vi "robotic arm main.vi"() -> ()   [LabVIEW 2019]
uses:
  <vilib>/myRIO/Instrument Drivers/Onboard IO/DIO/typedefs/DIO Reference.ctl
  <vilib>/myRIO/Common/Instrument Driver Framework/Utilities/typedefs/myRIO Generic Hardware Reference.ctl
  <vilib>/myRIO/Common/Instrument Driver Framework/Utilities/typedefs/Hardware Version Enum.ctl
  <vilib>/myRIO/Common/Instrument Driver Framework/Utilities/typedefs/myRIO v1.0 Reference.ctl
  <vilib>/myRIO/Common/Instrument Driver Framework/Utilities/typedefs/Generic FPGA Reference.ctl
  <vilib>/myRIO/Common/Instrument Driver Framework/myRIO v1.0/DIO/typedefs/DIO Channels List.ctl
  <vilib>/myRIO/Common/Instrument Driver Framework/myRIO v1.0/DIO/typedefs/DIO Channels Enum.ctl
  <vilib>/userdefined/High Color/nirio_resource_hc.ctl
  <vilib>/myRIO/Instrument Drivers/Onboard IO/PWM/typedefs/PWM Reference.ctl
  <vilib>/myRIO/Common/Instrument Driver Framework/myRIO v1.0/PWM/typedefs/PWM Channels Enum.ctl
  <vilib>/myRIO/Instrument Drivers/Onboard IO/PWM/typedefs/PWM Configuration.ctl
  <vilib>/myRIO/Common/Instrument Driver Framework/Utilities/vis/Is FPGA Ref Available.vi
  <vilib>/myRIO/Common/Instrument Driver Framework/myRIO v1.0/DIO/vis/myRIO v1.1 Open DIO.vi
  <vilib>/myRIO/Instrument Drivers/Onboard IO/DIO/vis/Read.vi
  <vilib>/myRIO/Common/Instrument Driver Framework/myRIO v1.0/PWM/vis/myRIO v1.1 Open PWM.vi
  <vilib>/myRIO/Instrument Drivers/Onboard IO/PWM/vis/Set Duty Cycle and Frequency.vi
  <vilib>/myRIO/Common/Instrument Driver Framework/Utilities/vis/Validate Channels.vi
  <vilib>/myRIO/Common/Instrument Driver Framework/myRIO v1.0/DIO/vis/myRIO v1.0 Reserve DIO.vi
  <vilib>/myRIO/Common/Instrument Driver Framework/myRIO v1.0/PWM/vis/myRIO v1.0 Reserve PWM.vi
  <vilib>/myRIO/Common/Instrument Driver Framework/myRIO v1.0/Resource Manager/vis/myRIO v1.0 Reserve Channel List.vi
  <vilib>/myRIO/Common/Instrument Driver Framework/myRIO v1.0/DIO/vis/myRIO v1.0 Build MUX Configuration DIO.vi
  <vilib>/myRIO/Common/Instrument Driver Framework/myRIO v1.0/PWM/vis/myRIO v1.0 Build MUX Configuration PWM.vi
  <vilib>/myRIO/Common/Instrument Driver Framework/myRIO v1.0/Resource Manager/vis/myRIO v1.0 Reserve Channel.vi
  <vilib>/myRIO/Common/Instrument Driver Framework/myRIO v1.0/Resource Manager/vis/myRIO v1.0 Unreserve Channel.vi
  <vilib>/myRIO/Common/Instrument Driver Framework/myRIO v1.0/Resource Manager/vis/myRIO v1.0 Create Configuration List.vi
  <vilib>/myRIO/Common/Instrument Driver Framework/myRIO v1.0/Resource Manager/vis/myRIO v1.0 Build Mutex Name.vi
  <vilib>/Utility/VariantDataType/GetNumericInfo.vi
  <vilib>/Utility/error.llb/Error Cluster From Error Code.vi
  <vilib>/myRIO/Common/Instrument Driver Framework/myRIO v1.0/myRIO v1.1 Open.vi
  <vilib>/myRIO/Common/Instrument Driver Framework/Utilities/vis/IO Manager.vi
  <vilib>/myRIO/Common/Instrument Driver Framework/Utilities/vis/Configuration Manager.vi
  <vilib>/myRIO/Common/Instrument Driver Framework/myRIO v1.0/Resource Manager/vis/myRIO v1.0 Configure IO.vi
  <vilib>/myRIO/Common/Instrument Driver Framework/myRIO v1.0/myRIO v1.0 Close.vi
  <vilib>/myRIO/Common/Instrument Driver Framework/myRIO v1.0/DIO/vis/myRIO v1.0 Read DIO.vi
  <vilib>/myRIO/Common/Instrument Driver Framework/myRIO v1.0/PWM/vis/myRIO v1.0 Write PWM.vi
  <vilib>/robotics/Kinematics/Generate Joint Trajectory (Int).vi
  <vilib>/myRIO/Express VI/Onboard IO/DI/DI Express VI.xnode
  <vilib>/myRIO/Instrument Drivers/Onboard IO/DIO/vis/myRIO DIO Open.xnode
  <vilib>/myRIO/Express VI/Onboard IO/PWM/PWM Express VI.xnode
  <vilib>/myRIO/Instrument Drivers/Onboard IO/PWM/vis/myRIO PWM Open.xnode
  <vilib>/robotics/Kinematics/NI_Kinematics.lvlib
  <vilib>/myRIO/Instrument Drivers/Onboard IO/PWM/PWM.lvlib
  <vilib>/myRIO/Instrument Drivers/Onboard IO/DIO/DIO.lvlib
panel:
  out "Position Sensor 2 (Pin 13)":bool
  out "Position Sensor 1 (Pin 11)":bool
  in  "Motion sequence or predefined?":bool
  out "State Number":i32
  in  "Motion sequence":T1
  in  "Control 6":dbl
  in  "Control 5":dbl
  in  "Control 4":dbl
  in  "Control 3":dbl
  in  "Control 2":dbl
  in  "Control 1":dbl
  out "1":dbl
  out "2":dbl
  out "3":dbl
  out "4":dbl
  out "5":dbl
  out "6":dbl
  in  "Start (Press time to start the action)":bool
  out "transposed array":dbl[][](array[numeric])
  out "start position":i32[](array[numeric])
  out "end position":i32[](array[numeric])
  out "joint position trajectory":dbl[][](array[numeric])
  out "Servo 1":dbl[](graph)
  out "Angle 1":dbl
  out "Angle 2":dbl
  out "Angle 3":dbl
  out "Angle 4":dbl
  out "Angle 5":dbl
  out "Angle 6":dbl
  out "Servo 2":dbl[](graph)
  out "Servo 3":dbl[](graph)
  out "Servo 4":dbl[](graph)
  out "Servo 5":dbl[](graph)
  out "Servo 6":dbl[](graph)
  in  "Switch mode":bool
  # "Agriculture Phenotyping Automation"
  # "EEM323 Robotics 2023\nMini Project Group 4\nLai Hong You, Justin Chia Vern Shuen, Thow Zhi An, Tiong Ji Kai"
  # "Control"
  # "Trajectory and Servos Status"
  # "State machine status"
  # "Motion \nSequence"
  # "Predefined"
  # "Sensor"
  # "Manual"
  # "Input"
  # "Output"
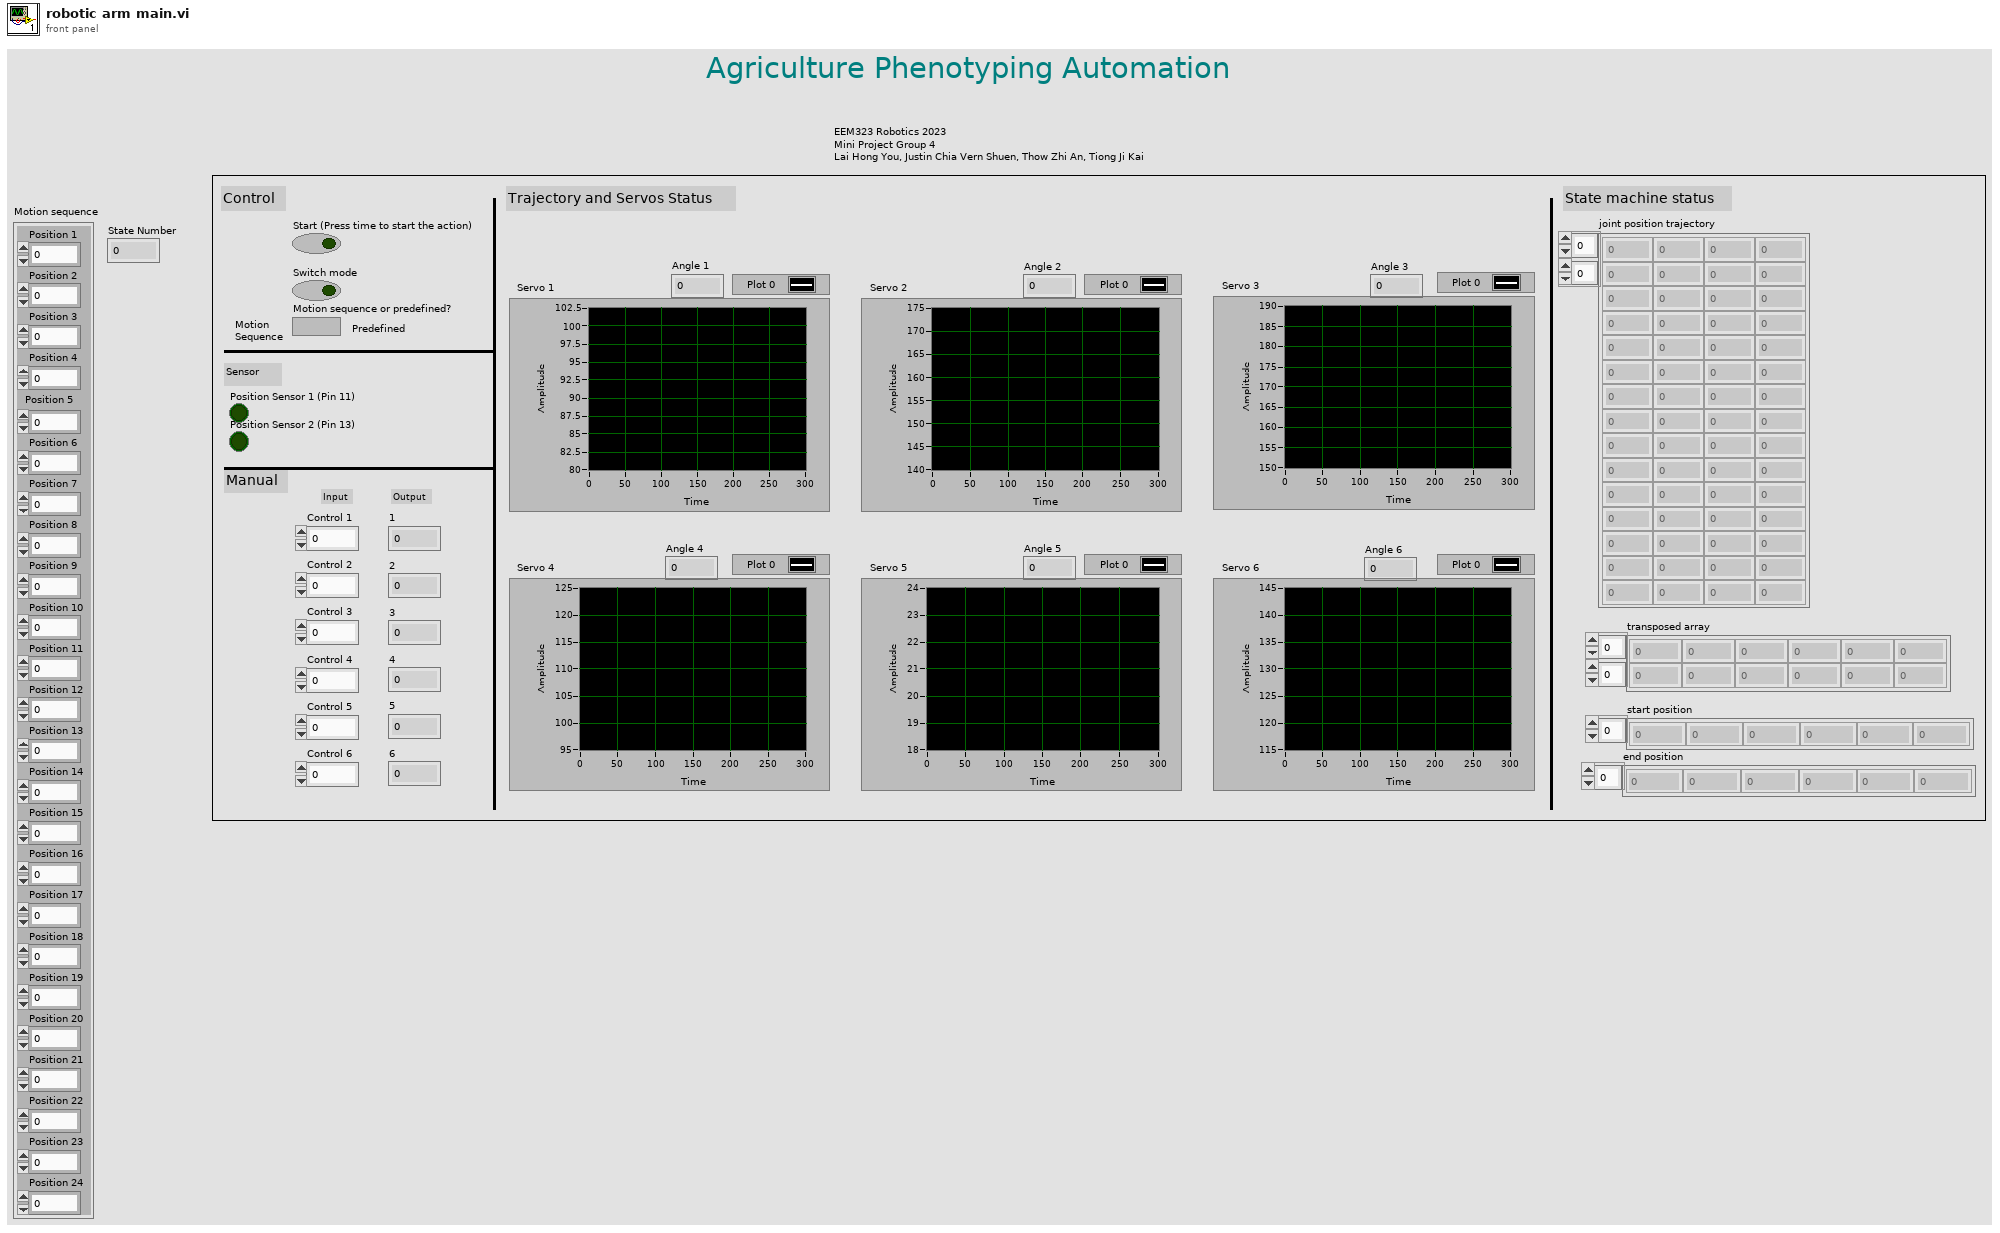
[diagram p1: front panel]
types:
  T1 = cluster{"Position 1":dbl, "Position 2":dbl, "Position 3":dbl, "Position 4":dbl, "Position 5":dbl, "Position 6":dbl, "Position 7":dbl, "Position 8":dbl, "Position 9":dbl, "Position 10":dbl, "Position 11":dbl, "Position 12":dbl, "Position 13":dbl, "Position 14":dbl, "Position 15":dbl, "Position 16":dbl, "Position 17":dbl, "Position 18":dbl, "Position 19":dbl, "Position 20":dbl, "Position 21":dbl, "Position 22":dbl, "Position 23":dbl, "Position 24":dbl}
  T2 = typedef "PWM.lvlib/PWM Reference.ctl" = cluster{"myRIO Reference":T3, "PWM Channels Enum":T7, "PWM Configuration":T8}
  T3 = typedef "myRIO Generic Hardware Reference.ctl" = cluster{"myRIO Model":T4, "myRIO Hardware Reference":T5}
  T4 = typedef "Hardware Version Enum.ctl" = enum16{"Unknown", "myRIO-1900", "myRIO-1950", "roboRIO", "NI ELVIS RIO CM", "ELVIS III"}
  T5 = typedef "myRIO v1.0 Reference.ctl" = cluster{"Generic FPGA Reference":T6, "Allow multiple opens":bool}
  T6 = typedef "Generic FPGA Reference.ctl" = refnum<k20>
  T7 = typedef "PWM Channels Enum.ctl" = enum16{"Not Connected", "C/PWM0", "C/PWM1", "A/PWM0", "A/PWM1", "A/PWM2", "A/PWM3", "A/PWM4", "A/PWM5", "A/PWM6", "A/PWM7", "A/PWM8", "A/PWM9", "A/PWM10", "A/PWM11", "A/PWM12", "A/PWM13", "A/PWM14", "A/PWM15", "A/PWM16", "A/PWM17", "A/PWM18", "A/PWM19", "B/PWM0", "B/PWM1", "B/PWM2", "B/PWM3", "B/PWM4", "B/PWM5", "B/PWM6", "B/PWM7", "B/PWM8", "B/PWM9", "B/PWM10", "B/PWM11", "B/PWM12", "B/PWM13", "B/PWM14", "B/PWM15", "B/PWM16", "B/PWM17", "B/PWM18", "B/PWM19", "PWM/PWM0", "PWM/PWM1", "PWM/PWM2", "PWM/PWM3", "PWM/PWM4", "PWM/PWM5", "PWM/PWM6", "PWM/PWM7", "PWM/PWM8", "PWM/PWM9"}
  T8 = typedef "PWM.lvlib/PWM Configuration.ctl" = cluster{"Frequency":dbl, "Duty Cycle":dbl}
  T9 = typedef "nirio_resource_hc.ctl" = tag
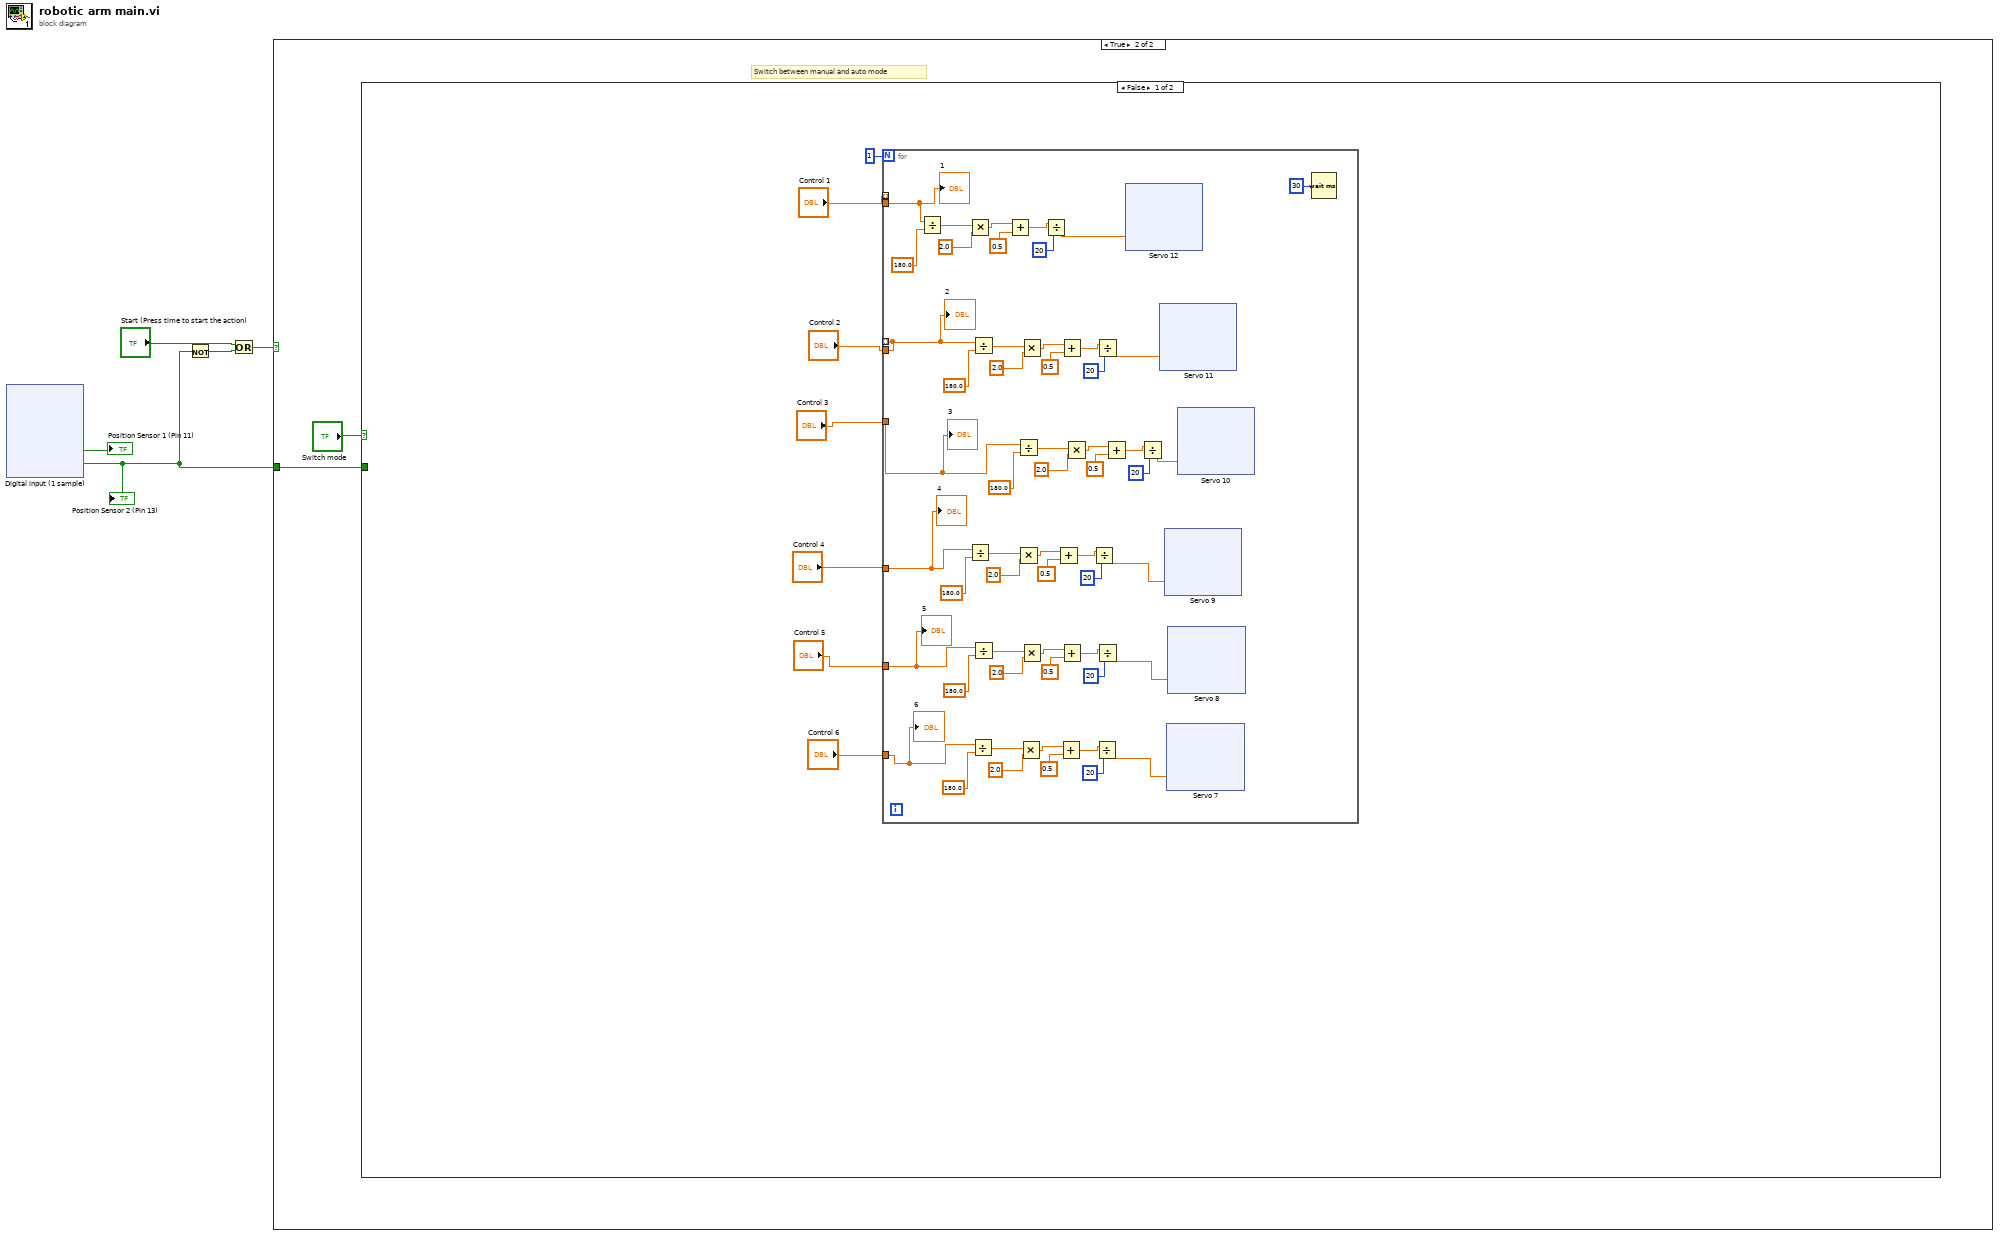
[diagram p0: block diagram]
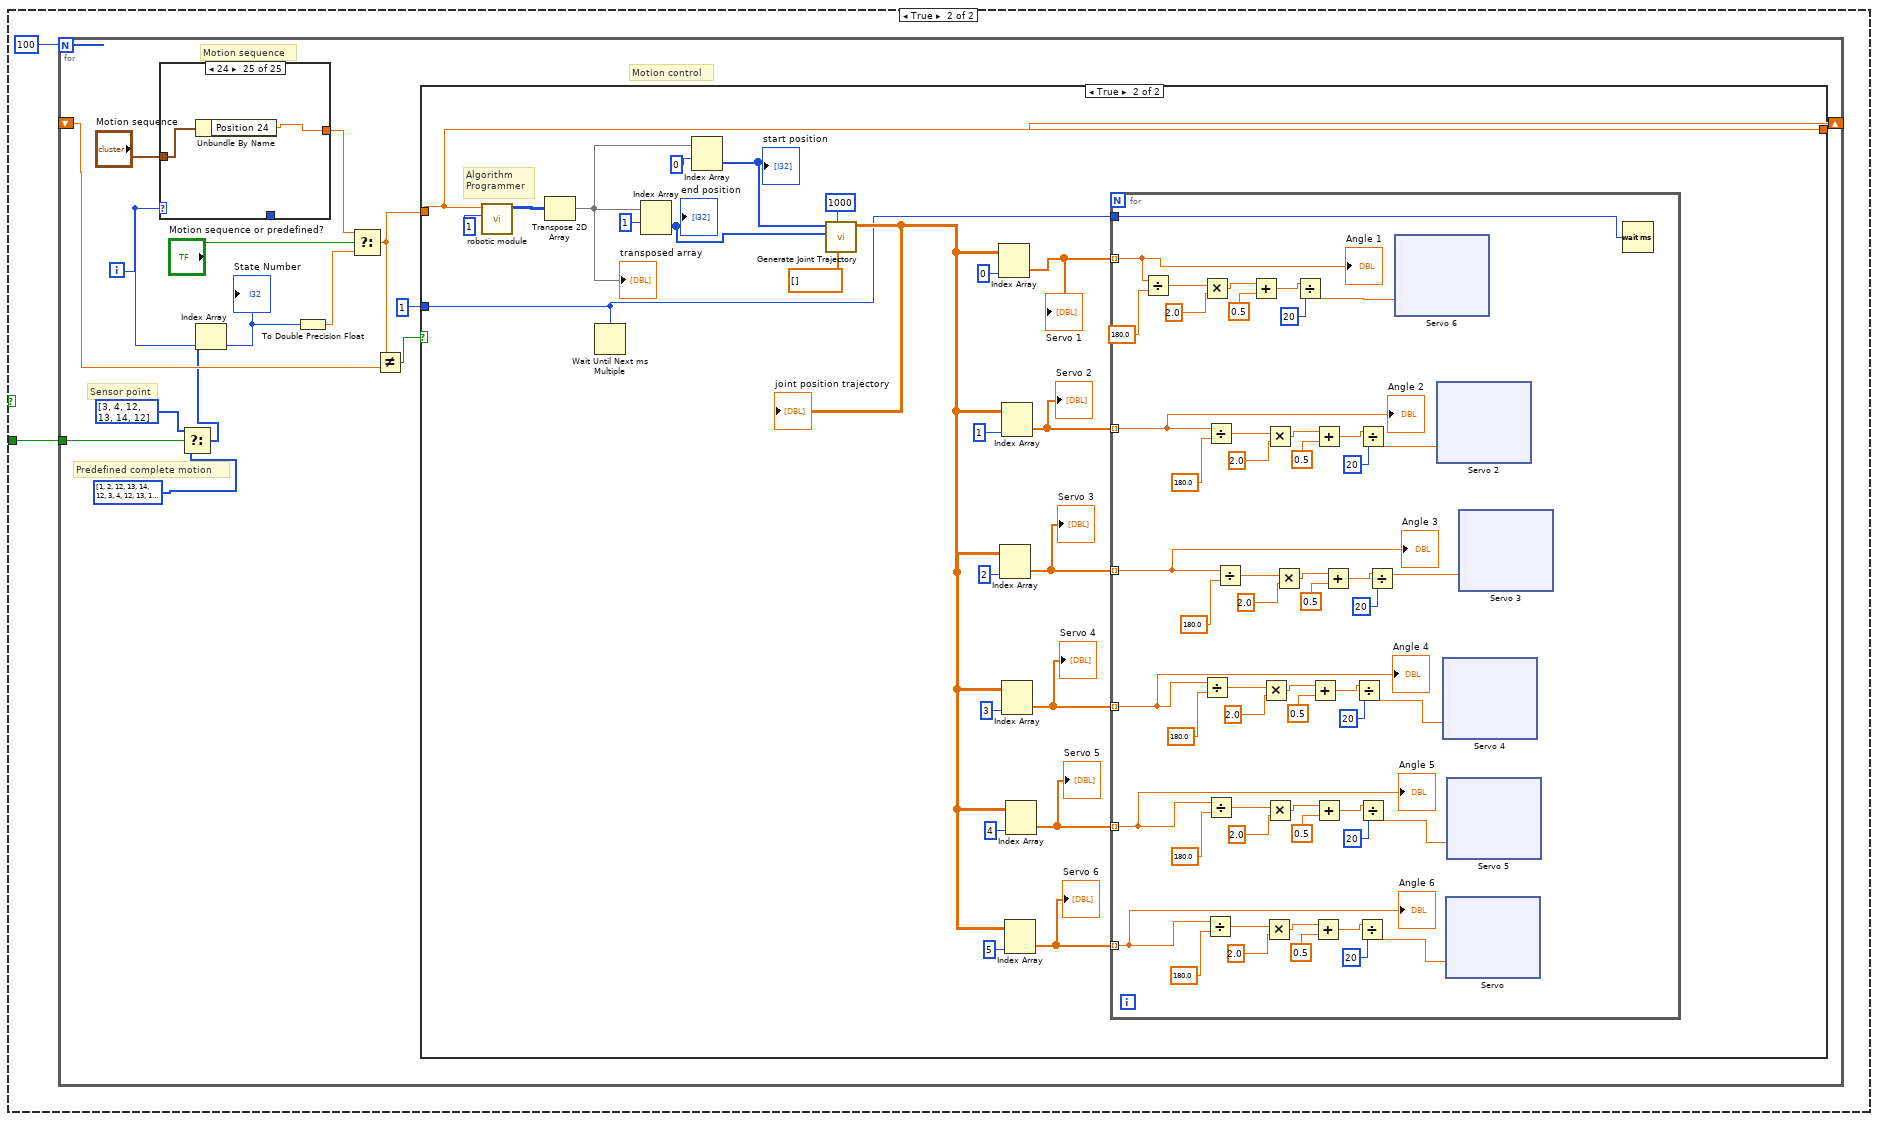
[diagram p3: hidden frame]
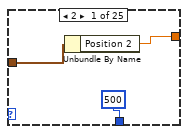
[diagram p4: hidden frame]
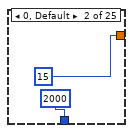
[diagram p5: hidden frame]
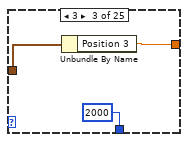
[diagram p6: hidden frame]
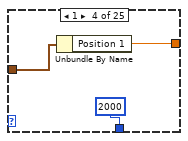
[diagram p7: hidden frame]
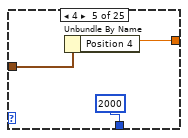
[diagram p8: hidden frame]
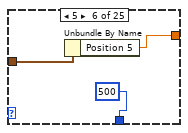
[diagram p9: hidden frame]
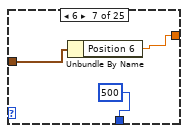
[diagram p10: hidden frame]
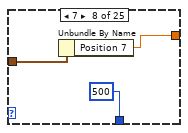
[diagram p11: hidden frame]
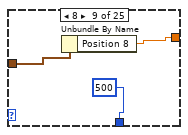
[diagram p12: hidden frame]
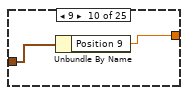
[diagram p13: hidden frame]
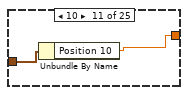
[diagram p14: hidden frame]
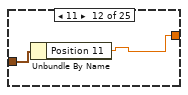
[diagram p15: hidden frame]
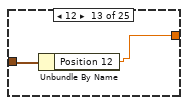
[diagram p16: hidden frame]
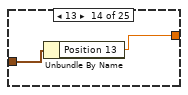
[diagram p17: hidden frame]
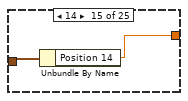
[diagram p18: hidden frame]
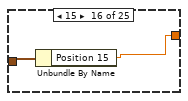
[diagram p19: hidden frame]
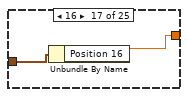
[diagram p20: hidden frame]
diagram:
  n1 = xnode "Digital input (1 sample)"() -> ("A/DIO0 (Pin 11)"=→"Position Sensor 1 (Pin 11)":bool, "A/DIO1 (Pin 13)"=w1:bool)  [unwired: 1 in, 1 out]
  "Position Sensor 2 (Pin 13)" <- w1
  n2 = Not(x=w1) -> (.not. x?=w4:bool)
  n3 = Or(x="Start (Press time to start the action)", y=w4) -> (x .or. y?=w3:bool)
  n4 = case shown="True" w3 {
    tunnel: w1 -> [_ w6]
    frame False {
    }
    frame True {
      # "Switch between manual and auto mode"
      n5 = case shown="False" "Switch mode" {
        tunnel: w6 -> [_ w280]
        frame False {
          n6 = for {
            N: 1 -> [_]
            tunnel: [w17] -> _ mode=indexing
            tunnel: [w16] -> _ mode=indexing
            tunnel: "Control 3" -> [w21]
            tunnel: "Control 4" -> [w20]
            tunnel: "Control 5" -> [w19]
            tunnel: "Control 1" -> [w17]
            tunnel: "Control 2" -> [w16]
            tunnel: "Control 6" -> [w15]
            n7 = Divide(x=w17, y=180.0) -> (x/y=w64:dbl)
            n8 = Multiply(x=w64, y=2.0) -> (x*y=w68:dbl)
            n9 = Divide(x=w20, y=180.0) -> (x/y=w40:dbl)
            n10 = Divide(x=w15, y=180.0) -> (x/y=w24:dbl)
            n11 = Divide(x=w16, y=180.0) -> (x/y=w56:dbl)
            n12 = Divide(x=w19, y=180.0) -> (x/y=w35:dbl)
            n13 = Add(x=w68, y=0.5) -> (x+y=w66:dbl)
            n14 = Divide(x=w21, y=180.0) -> (x/y=w51:dbl)
            n15 = Multiply(x=w40, y=2.0) -> (x*y=w44:dbl)
            n16 = Multiply(x=w24, y=2.0) -> (x*y=w28:dbl)
            n17 = Multiply(x=w56, y=2.0) -> (x*y=w60:dbl)
            n18 = Multiply(x=w35, y=2.0) -> (x*y=w31:dbl)
            n19 = Divide(x=w66, y=20) -> (x/y=w63:dbl)
            n20 = Add(x=w44, y=0.5) -> (x+y=w42:dbl)
            n21 = Add(x=w28, y=0.5) -> (x+y=w26:dbl)
            n22 = Add(x=w60, y=0.5) -> (x+y=w58:dbl)
            n23 = Add(x=w31, y=0.5) -> (x+y=w33:dbl)
            n24 = Multiply(x=w51, y=2.0) -> (x*y=w47:dbl)
            n25 = Divide(x=w42, y=20) -> (x/y=w39:dbl)
            n26 = Divide(x=w26, y=20) -> (x/y=w23:dbl)
            n27 = Divide(x=w58, y=20) -> (x/y=w55:dbl)
            n28 = Divide(x=w33, y=20) -> (x/y=w36:dbl)
            n29 = Add(x=w47, y=0.5) -> (x+y=w49:dbl)
            n30 = xnode "Servo 12"("Duty Cycle"=w63) -> ()  [unwired: 1 in, 1 out]
            n31 = Divide(x=w49, y=20) -> (x/y=w52:dbl)
            n32 = xnode "Servo 11"("Duty Cycle"=w55) -> ()  [unwired: 1 in, 1 out]
            n33 = xnode "Servo 9"("Duty Cycle"=w39) -> ()  [unwired: 1 in, 1 out]
            n34 = xnode "Servo 7"("Duty Cycle"=w23) -> ()  [unwired: 1 in, 1 out]
            n35 = xnode "Servo 8"("Duty Cycle"=w36) -> ()  [unwired: 1 in, 1 out]
            n36 = xnode "Servo 10"("Duty Cycle"=w52) -> ()  [unwired: 1 in, 1 out]
            n37 = Wait (ms)(milliseconds to wait=u32 30) -> ()  [unwired: 1 out]
            "1" <- w17
            "2" <- w16
            "3" <- w21
            "4" <- w20
            "5" <- w19
            "6" <- w15
          }
        }
        frame True {
          n38 = for {
            N: 100 -> [_]
            shift-right: [w296] -> _
            shift-left: _ -> [w292]
            tunnel: w280 -> [w283]
            i -> [w286]
            # "Sensor point"
            # "Predefined complete motion"
            # "Motion sequence"
            # "Motion control"
            n39 = case shown="24" w286 {
              tunnel: "Motion sequence" -> [w299 _ w304 w307 w309 w313 w315 w319 w320 w323 w325 w327 w329 w331 w334 w335 w337 w339 w341 w343 w345 w347 w349 w352 w353]
              tunnel: [w298 15 w303 w306 w310 w312 w316 w318 w321 w324 w326 w328 w330 w332 w333 w336 w338 w340 w342 w344 w346 w348 w350 w351 w354] -> w294
              tunnel: [u32 500 ("millisecond multiple") u32 2000 ("millisecond multiple") u32 2000 ("millisecond multiple") u32 2000 ("millisecond multiple") u32 2000 ("millisecond multiple") u32 500 ("millisecond multiple") u32 500 ("millisecond multiple") u32 500 ("millisecond multiple") u32 500 ("millisecond multiple") _ _ _ _ _ _ _ _ _ _ _ _ _ _ _ _] -> _
              frame 2 {
                n40 = Unbundle By Name(w299) -> ("Position 2"=w298:dbl)
              }
              frame 0, Default {
              }
              frame 3 {
                n41 = Unbundle By Name(w304) -> ("Position 3"=w303:dbl)
              }
              frame 1 {
                n42 = Unbundle By Name(w307) -> ("Position 1"=w306:dbl)
              }
              frame 4 {
                n43 = Unbundle By Name(w309) -> ("Position 4"=w310:dbl)
              }
              frame 5 {
                n44 = Unbundle By Name(w313) -> ("Position 5"=w312:dbl)
              }
              frame 6 {
                n45 = Unbundle By Name(w315) -> ("Position 6"=w316:dbl)
              }
              frame 7 {
                n46 = Unbundle By Name(w319) -> ("Position 7"=w318:dbl)
              }
              frame 8 {
                n47 = Unbundle By Name(w320) -> ("Position 8"=w321:dbl)
              }
              frame 9 {
                n48 = Unbundle By Name(w323) -> ("Position 9"=w324:dbl)
              }
              frame 10 {
                n49 = Unbundle By Name(w325) -> ("Position 10"=w326:dbl)
              }
              frame 11 {
                n50 = Unbundle By Name(w327) -> ("Position 11"=w328:dbl)
              }
              frame 12 {
                n51 = Unbundle By Name(w329) -> ("Position 12"=w330:dbl)
              }
              frame 13 {
                n52 = Unbundle By Name(w331) -> ("Position 13"=w332:dbl)
              }
              frame 14 {
                n53 = Unbundle By Name(w334) -> ("Position 14"=w333:dbl)
              }
              frame 15 {
                n54 = Unbundle By Name(w335) -> ("Position 15"=w336:dbl)
              }
              frame 16 {
                n55 = Unbundle By Name(w337) -> ("Position 16"=w338:dbl)
              }
              frame 17 {
                n56 = Unbundle By Name(w339) -> ("Position 17"=w340:dbl)
              }
              frame 18 {
                n57 = Unbundle By Name(w341) -> ("Position 18"=w342:dbl)
              }
              frame 19 {
                n58 = Unbundle By Name(w343) -> ("Position 19"=w344:dbl)
              }
              frame 20 {
                n59 = Unbundle By Name(w345) -> ("Position 20"=w346:dbl)
              }
              frame 21 {
                n60 = Unbundle By Name(w347) -> ("Position 21"=w348:dbl)
              }
              frame 22 {
                n61 = Unbundle By Name(w349) -> ("Position 22"=w350:dbl)
              }
              frame 23 {
                n62 = Unbundle By Name(w352) -> ("Position 23"=w351:dbl)
              }
              frame 24 {
                n63 = Unbundle By Name(w353) -> ("Position 24"=w354:dbl)
              }
            }
            n64 = Select(t=i32[] [3, 4, 12, 13, 14, 12] ("array"), s=w283, f=i32[] [1, 2, 12, 13, 14, 12, 3, 4, 12, 13, 14, 12, 5, 6, 12, 13, 14, 12, 7, 8, 9, 10, 11, 15]) -> (s? t:f=w282:i32[])
            n65 = Index Array(array=w282, index=w286) -> (element=w288:i32)
            "State Number" <- w288
            n66 = To Double Precision Float(number=w288) -> (double precision float=w287:dbl)
            n67 = Select(t=w294, s="Motion sequence or predefined?", f=w287) -> (s? t:f=w289:dbl)
            n68 = Not Equal?(x=w289, y=w292) -> (x != y?=w290:bool)
            n69 = case shown="True" w290 {
              tunnel: w289 -> [w355 w374]
              tunnel: [w355 w374] -> w296
              tunnel: u32 1 ("millisecond multiple") -> [_ w358]
              frame False {
              }
              frame True {
                # "Algorithm\nProgrammer"
                n70 = call "robotic module.vi"("Repeat (MUST BE 1)"=1, "motion type"=w374) -> ("array"=w378:i32[][])  [unwired: 9 in]
                n71 = Transpose 2D Array(2D array=w378) -> (transposed array=w376:i32[][])
                "transposed array" <- w376
                n72 = Wait Until Next ms Multiple(millisecond multiple=w358) -> ()  [unwired: 1 out]
                n73 = Index Array(array=w376, index (row)=1) -> (element=w356:i32[])  [unwired: 1 in]
                "end position" <- w356
                n74 = Index Array(array=w376, index (row)=0) -> (element=w357:i32[])  [unwired: 1 in]
                "start position" <- w357
                n75 = call-poly <vilib>:"Generate Joint Trajectory.vi"("start joint velocities"=dbl[] [], "intermediate points"=1000, "end joint positions"=w356, "start joint positions"=w357) -> ("joint position trajectory"=w359:dbl[][])  [unwired: 4 in, 3 out]
                "joint position trajectory" <- w359
                n76 = Index Array(array=w359, index (col)=0 ("disabled index (col)")) -> (element=w371:dbl[])  [unwired: 1 in]
                "Servo 1" <- w371
                n77 = Index Array(array=w359, index (col)=2) -> (element=w367:dbl[])  [unwired: 1 in]
                "Servo 3" <- w367
                n78 = Index Array(array=w359, index (col)=1 ("disabled index (col)")) -> (element=w366:dbl[])  [unwired: 1 in]
                "Servo 2" <- w366
                n79 = Index Array(array=w359, index (col)=3) -> (element=w364:dbl[])  [unwired: 1 in]
                "Servo 4" <- w364
                n80 = Index Array(array=w359, index (col)=5) -> (element=w360:dbl[])  [unwired: 1 in]
                "Servo 6" <- w360
                n81 = Index Array(array=w359, index (col)=4) -> (element=w363:dbl[])  [unwired: 1 in]
                "Servo 5" <- w363
                n82 = for {
                  tunnel: w371 -> [w386] mode=indexing
                  tunnel: w366 -> [w385] mode=indexing
                  tunnel: w367 -> [w384] mode=indexing
                  tunnel: w364 -> [w383] mode=indexing
                  tunnel: w363 -> [w382] mode=indexing
                  tunnel: w360 -> [w381] mode=indexing
                  tunnel: w358 -> [w380]
                  n83 = Divide(x=w386, y=180.0) -> (x/y=w429:dbl)
                  n84 = Multiply(x=w429, y=2.0) -> (x*y=w433:dbl)
                  n85 = Divide(x=w383, y=180.0) -> (x/y=w405:dbl)
                  n86 = Divide(x=w381, y=180.0) -> (x/y=w389:dbl)
                  n87 = Divide(x=w385, y=180.0) -> (x/y=w421:dbl)
                  n88 = Divide(x=w382, y=180.0) -> (x/y=w400:dbl)
                  n89 = Divide(x=w384, y=180.0) -> (x/y=w416:dbl)
                  n90 = Add(x=w433, y=0.5) -> (x+y=w431:dbl)
                  n91 = Multiply(x=w405, y=2.0) -> (x*y=w409:dbl)
                  n92 = Multiply(x=w389, y=2.0) -> (x*y=w393:dbl)
                  n93 = Multiply(x=w421, y=2.0) -> (x*y=w425:dbl)
                  n94 = Multiply(x=w400, y=2.0) -> (x*y=w396:dbl)
                  n95 = Multiply(x=w416, y=2.0) -> (x*y=w412:dbl)
                  n96 = Divide(x=w431, y=20) -> (x/y=w428:dbl)
                  n97 = Add(x=w409, y=0.5) -> (x+y=w407:dbl)
                  n98 = Add(x=w393, y=0.5) -> (x+y=w391:dbl)
                  n99 = Add(x=w425, y=0.5) -> (x+y=w423:dbl)
                  n100 = Add(x=w396, y=0.5) -> (x+y=w398:dbl)
                  n101 = Add(x=w412, y=0.5) -> (x+y=w414:dbl)
                  n102 = Divide(x=w407, y=20) -> (x/y=w404:dbl)
                  n103 = Divide(x=w391, y=20) -> (x/y=w388:dbl)
                  n104 = Divide(x=w423, y=20) -> (x/y=w420:dbl)
                  n105 = Divide(x=w398, y=20) -> (x/y=w401:dbl)
                  n106 = Divide(x=w414, y=20) -> (x/y=w417:dbl)
                  n107 = xnode "Servo 6"("Duty Cycle"=w428) -> ()  [unwired: 1 in, 1 out]
                  n108 = xnode "Servo 2"("Duty Cycle"=w420) -> ()  [unwired: 1 in, 1 out]
                  n109 = xnode "Servo 4"("Duty Cycle"=w404) -> ()  [unwired: 1 in, 1 out]
                  n110 = xnode "Servo"("Duty Cycle"=w388) -> ()  [unwired: 1 in, 1 out]
                  n111 = xnode "Servo 5"("Duty Cycle"=w401) -> ()  [unwired: 1 in, 1 out]
                  n112 = xnode "Servo 3"("Duty Cycle"=w417) -> ()  [unwired: 1 in, 1 out]
                  n113 = Wait (ms)(milliseconds to wait=w380) -> ()  [unwired: 1 out]
                  "Angle 1" <- w386
                  "Angle 2" <- w385
                  "Angle 3" <- w384
                  "Angle 4" <- w383
                  "Angle 5" <- w382
                  "Angle 6" <- w381
                }
              }
            }
          }
        }
      }
    }
  }
